vi "Expand the Compact Array.vi"(8 "error in (no error)":errorcluster, 10 "Arr Refnum":refnum<vi>, 11 "File Refnum":T1) -> (0 "error out":errorcluster, 2 "dup Arr Refnum":refnum<vi>, 3 "dup File Refnum":T1)   [LabVIEW 2013]
uses:
  <vilib>/Utility/config.llb/Config Data RefNum.ctl
  control/OD Entry.ctl
  control/Object Type.ctl
  control/Data Type.ctl
  control/Access Type.ctl
  control/OD Cateory.ctl
  <vilib>/Utility/config.llb/NI_LVConfig.lvlib
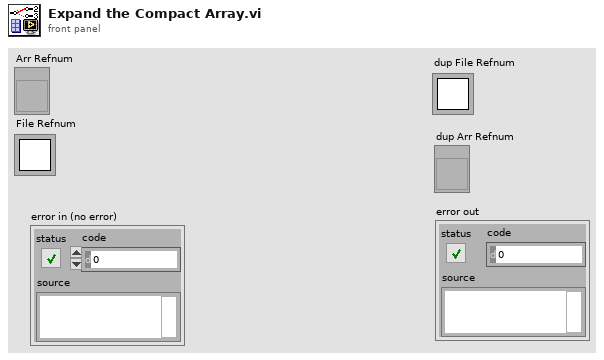
[diagram p1: front panel]
types:
  T1 = typedef "NI_LVConfig.lvlib/Config Data RefNum.ctl" = refnum<k1>
  T2 = typedef "OD Entry.ctl" = cluster{"index":u16, "sub-index":u8, "Level":u8, "ObjectType":T3, "DataType":T4, "ParameterName":string, "LowLimit":string, "HighLimit":string, "AccessType":T5, "DefaultValue":string, "PDOMapping":bool, "SubNumber":u8, "ObjFlags":u32, "Category":T6}
  T3 = typedef "Object Type.ctl" = u16
  T4 = typedef "Data Type.ctl" = u16
  T5 = typedef "Access Type.ctl" = u16
  T6 = typedef "OD Cateory.ctl" = enum16{"Mandatory", "Optional", "Manufacturer", ""}
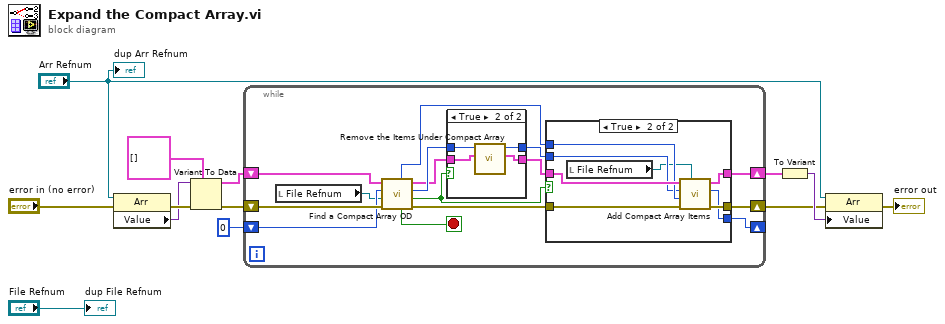
[diagram p0: block diagram]
diagram:
  n1 = property class="Arr"(reference="Arr Refnum", error in="error in (no error)") -> (error out=w12:errorcluster, "Value"=w11:variant)  [unwired: 1 out]
  n2 = Variant To Data(error in=w12, type=T2[] [], Variant=w11) -> (data=w8:T2[], error out=w9:errorcluster)
  n3 = while {
    shift-right: [w17] -> w5
    shift-left: w9 -> [w28]
    shift-right: [w18] -> w7
    shift-left: w8 -> [w26]
    shift-right: [w25] -> _
    shift-left: 0 -> [w27]
    stop <- w14 stop-if-true
    n4 = local read "File Refnum"() -> (w15:T1)
    n5 = call "Find a Compact Array OD.vi"("error in"=w28, "File Refnum"=w15, "Index"=w27, "ODs"=w26) -> ("error out"=w22:errorcluster, "Found?"=w19:bool, "Next Index"=w24:i32, "dup ODs"=w23:T2[], "Stop?"=w14:bool, "Count"=w16:u8)  [unwired: 2 in]
    n6 = case shown="True" w19 {
      tunnel: w23 -> [w41 w45]
      tunnel: [w41 w42] -> w20
      tunnel: w24 -> [w40 w44]
      tunnel: [w40 w43] -> w21
      frame False {
      }
      frame True {
        n7 = call "Remove the Items Under Compact Array.vi"("ODs in"=w45, "Index"=w44) -> ("ODs out"=w42:T2[], "Next Index"=w43:i32)  [unwired: 8 in]
      }
    }
    n8 = case shown="True" w19 {
      tunnel: w20 -> [w31 w37]
      tunnel: [w31 w36] -> w18
      tunnel: w22 -> [w30 w39]
      tunnel: [w30 w38] -> w17
      tunnel: w21 -> [w29 w34]
      tunnel: w16 -> [_ w35]
      tunnel: [w29 w33] -> w25
      frame False {
      }
      frame True {
        n9 = local read "File Refnum"() -> (w32:T1)
        n10 = call "Add Compact Array Items.vi"("File Refnum"=w32, "error in"=w39, "Count"=w35, "Index"=w34, "ODs in"=w37) -> ("error out"=w38:errorcluster, "Next Index"=w33:i32, "ODs out"=w36:T2[])  [unwired: 4 in]
      }
    }
  }
  n11 = To Variant(anything=w7) -> (Variant=w6:variant)
  n12 = property class="Arr"(reference="Arr Refnum", error in=w5, "Value"=w6) -> (error out=→"error out":errorcluster)  [unwired: 1 out]
  "dup Arr Refnum" <- "Arr Refnum"
  "dup File Refnum" <- "File Refnum"
